vi "Priority.vi"(8 "error in (no error)":errorcluster, 11 "FileNotFoundException in":refnum<class "FileNotFoundException.lvclass">) -> (0 "error out":errorcluster, 2 "Priority":u16, 3 "FileNotFoundException out":refnum<class "FileNotFoundException.lvclass">)   [LabVIEW 2020, in "HTTP Server.lvlib" / "FileNotFoundException.lvclass"]
uses:
  FileNotFoundException.lvclass
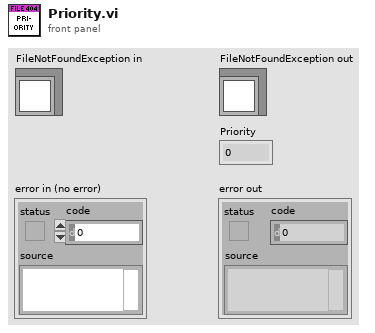
[diagram p1: front panel]
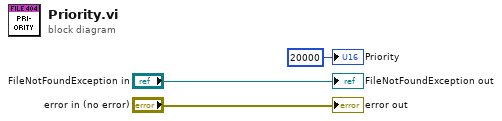
[diagram p0: block diagram]
diagram:
  "error out" <- "error in (no error)"
  "FileNotFoundException out" <- "FileNotFoundException in"
  "Priority" <- u16 20000 ("Priority")
